vi "Calibrate.vi"(1 "nano handle":i32, 2 "Changing Axis":bool, 3 "tirf handle":i32) -> (0 "cal":dbl)   [LabVIEW 2019]
uses:
  Madlib.dll
  <vilib>/Analysis/NI_AALPro.lvlib
panel:
  out "DAC":cluster{i32[], dbl[]}(graph)
  out "XY Voltage":cluster{i32[], dbl[]}(graph)
  out "Running":bool
  in  "Display":bool=TRUE
  in  "Averages":i32=20 min=1
  # "X"
  # "Y"
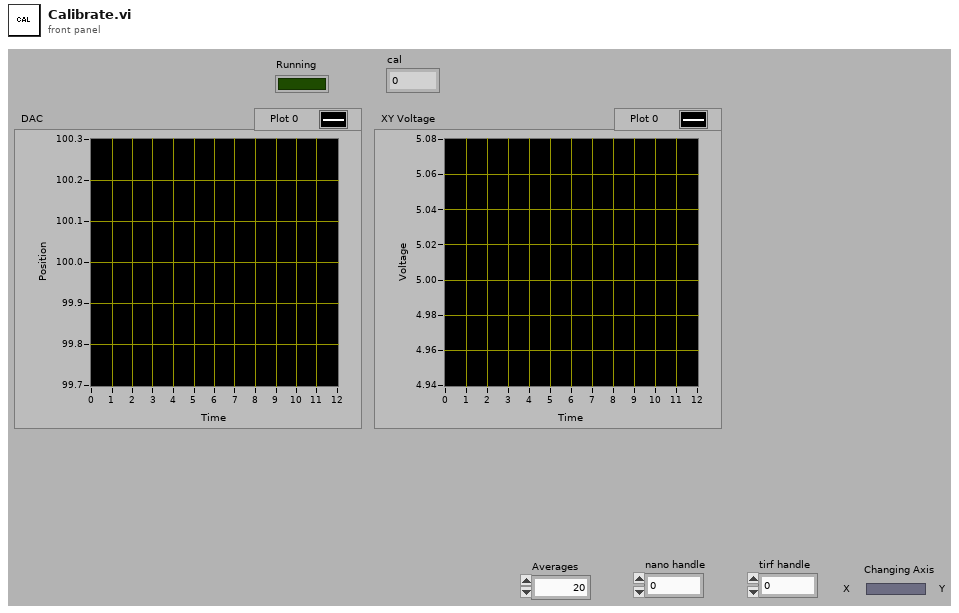
[diagram p1: front panel]
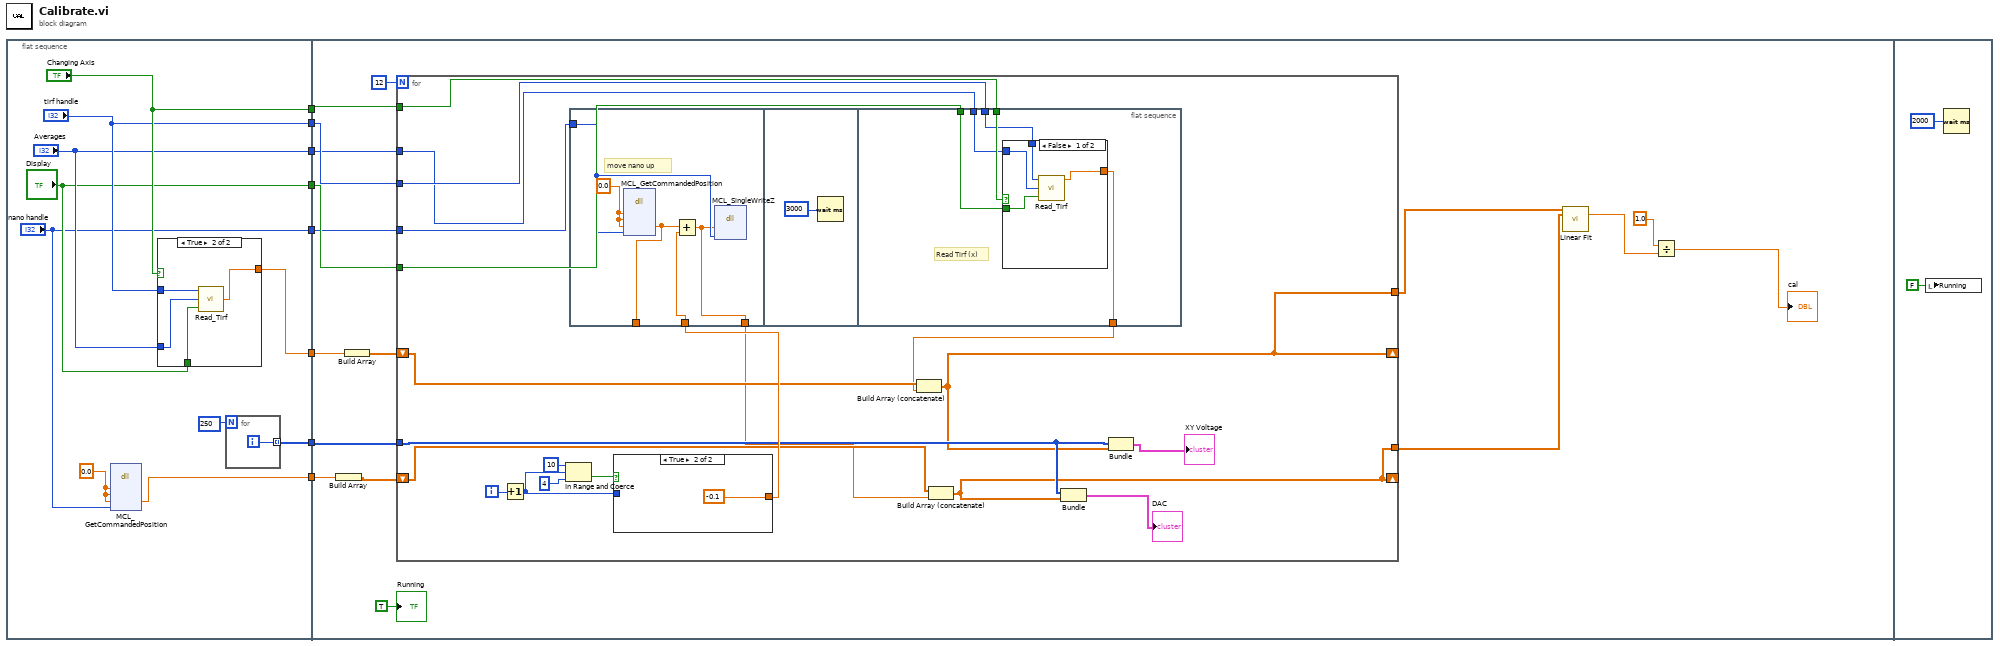
[diagram p0: block diagram]
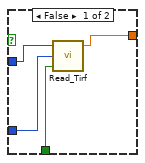
[diagram p2: hidden frame]
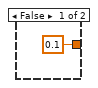
[diagram p3: hidden frame]
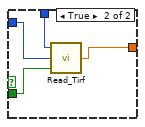
[diagram p4: hidden frame]
diagram:
  n1 = flat-sequence {
    tunnel: [w17] -> w8
    tunnel: [w16] -> w7
    tunnel: ["Changing Axis"] -> w6
    tunnel: ["tirf handle"] -> w5
    tunnel: ["Averages"] -> w4
    tunnel: ["Display"] -> w3
    tunnel: ["nano handle"] -> w2
    tunnel: [w9] -> w1
    tunnel: w8 -> [w42]
    tunnel: w7 -> [w37]
    tunnel: w6 -> [w35]
    tunnel: w5 -> [w34]
    tunnel: w4 -> [w33]
    tunnel: w3 -> [w32]
    tunnel: w2 -> [w31]
    tunnel: w1 -> [w29]
    frame #0 {
      w10 = 0.0 ("commandX")
      n2 = dll-call lib="E:/DevHardSoftware/MMicroscopy/HardwareAdapter/Stages/Dependencies/Madlib.dll" fn="MCL_GetCommandedPosition" ("MCL_SingleReadN")("commandX"=w10, "commandY"=w10, "commandZ"=w10, "handle"="nano handle") -> ("commandZ"=w9:dbl)  [unwired: 5 in, 4 out]
      n3 = case shown="True" "Changing Axis" {
        tunnel: [w22 w26] -> w16
        tunnel: "tirf handle" -> [w21 w23]
        tunnel: "Averages" -> [w20 w24]
        tunnel: "Display" -> [w19 w25]
        frame False {
          n4 = call "Read_Tirf.vi"("Display"=w19, "Averages"=w20, "Tirf-Handle"=w21) -> ("coerced(x)"=w22:dbl)  [unwired: 2 out]
        }
        frame True {
          n5 = call "Read_Tirf.vi"("Display"=w25, "Averages"=w24, "Tirf-Handle"=w23) -> ("coerced(y)"=w26:dbl)  [unwired: 2 out]
        }
      }
      n6 = for {
        N: 250 -> [_]
        tunnel: [w27] -> w17 mode=indexing
        i -> [w27]
      }
    }
    frame #1 {
      n7 = Build Array(w29) -> (w30:dbl[])
      n8 = Build Array(w37) -> (w36:dbl[])
      n9 = for {
        N: 12 -> [_]
        shift-right: [w52] -> _
        shift-left: w36 -> [w63]
        tunnel: w42 -> [w59]
        shift-right: [w54] -> _
        shift-left: w30 -> [w61]
        tunnel: [w54] -> w40
        tunnel: [w52] -> w41
        tunnel: w35 -> [w50]
        tunnel: w34 -> [w49]
        tunnel: w33 -> [w48]
        tunnel: w32 -> [w47]
        tunnel: w31 -> [w46]
        i -> [w53]
        n10 = Increment(x=w53) -> (x+1=w58:i32)
        n11 = In Range and Coerce(upper limit=10, x=w58, lower limit=4) -> (In Range?=w55:bool)  [unwired: 1 out]
        n12 = flat-sequence {
          tunnel: w64 -> [w70]
          tunnel: [w69] -> _
          tunnel: [w68] -> w45
          tunnel: w46 -> [w71]
          tunnel: [w77] -> w51
          tunnel: w50 -> [w76]
          tunnel: w49 -> [w75]
          tunnel: w48 -> [w74]
          tunnel: w47 -> [w73]
          frame #0 {
            w67 = 0.0 ("commandX")
            # "move nano up"
            n13 = dll-call lib="E:/DevHardSoftware/MMicroscopy/HardwareAdapter/Stages/Dependencies/Madlib.dll" fn="MCL_GetCommandedPosition" ("MCL_SingleReadN")("commandX"=w67, "commandY"=w67, "commandZ"=w67, "handle"=w71) -> ("commandZ"=w69:dbl)  [unwired: 5 in, 4 out]
            n14 = Add(x=w69, y=w70) -> (x+y=w68:dbl)
            n15 = dll-call lib="E:/DevHardSoftware/MMicroscopy/HardwareAdapter/Stages/Dependencies/Madlib.dll" fn="MCL_SingleWriteZ"("position"=w68, "handle"=w71) -> ()  [unwired: 3 in, 5 out]
          }
          frame #1 {
            n16 = Wait (ms)(milliseconds to wait=u32 3000) -> ()  [unwired: 1 out]
          }
          frame #2 {
            # "Read Tirf (x)"
            n17 = case shown="False" w76 {
              tunnel: [w81 w85] -> w77
              tunnel: w75 -> [w80 w84]
              tunnel: w74 -> [w79 w83]
              tunnel: w73 -> [w78 w82]
              frame False {
                n18 = call "Read_Tirf.vi"("Display"=w78, "Averages"=w79, "Tirf-Handle"=w80) -> ("coerced(x)"=w81:dbl)  [unwired: 2 out]
              }
              frame True {
                n19 = call "Read_Tirf.vi"("Display"=w82, "Averages"=w83, "Tirf-Handle"=w84) -> ("coerced(y)"=w85:dbl)  [unwired: 2 out]
              }
            }
          }
        }
        n20 = case shown="True" w55 {
          tunnel: w58 -> [_ _]
          tunnel: [0.1 ("f") -0.1 ("f")] -> w64
          frame False {
          }
          frame True {
          }
        }
        n21 = Build Array (concatenate)(w63, w51) -> (w52:dbl[])
        n22 = Build Array (concatenate)(w61, w45) -> (w54:dbl[])
        n23 = Bundle(w59, w54) -> (→"DAC":cluster{i32[], dbl[]})  [unwired: 1 in]
        n24 = Bundle(w59, w52) -> (→"XY Voltage":cluster{i32[], dbl[]})  [unwired: 1 in]
      }
      n25 = call <vilib>:"Linear Fit.vi"("Y"=w41, "X"=w40) -> ("slope"=w38:dbl)  [unwired: 9 in, 4 out]
      n26 = Divide(x=1.0, y=w38) -> (x/y=→"cal":dbl)
      "Running" <- TRUE ("Running")
    }
    frame #2 {
      n27 = local write "Running"(FALSE ("Running")) -> ()
      n28 = Wait (ms)(milliseconds to wait=u32 2000) -> ()  [unwired: 1 out]
    }
  }
